vi "Main.vi"(4 "States":T1(ring), 5 "name":string="Name", 6 "error in":errorcluster, 8 "elemint in":variant, 9 "queue in":refnum<queue>) -> (0 "error out":errorcluster, 2 "element out":variant, 3 "queue out":refnum<queue>)   [LabVIEW 2010]
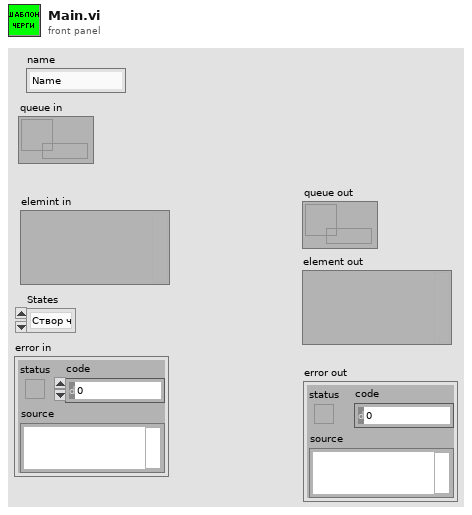
[diagram p1: front panel]
types:
  T1 = enum16{"Створ ч", "Зап на поч", "Зап на кін", "Зчит", "Очищ", "Видал"}
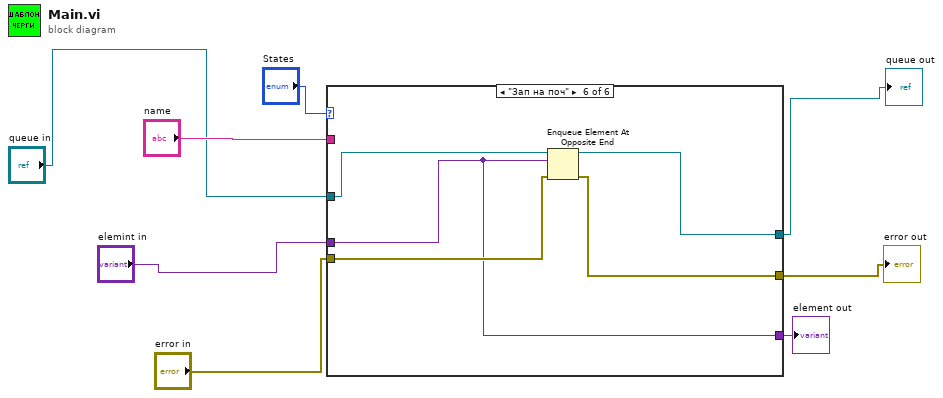
[diagram p0: block diagram]
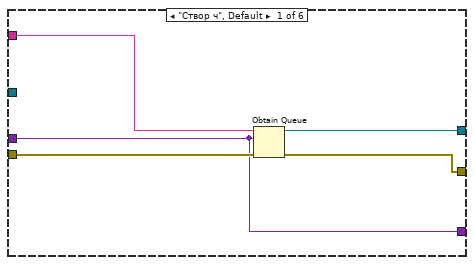
[diagram p2: hidden frame]
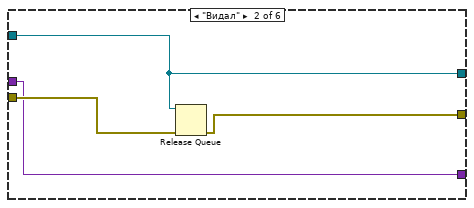
[diagram p3: hidden frame]
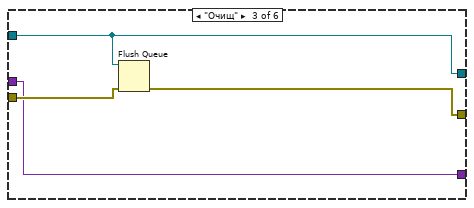
[diagram p4: hidden frame]
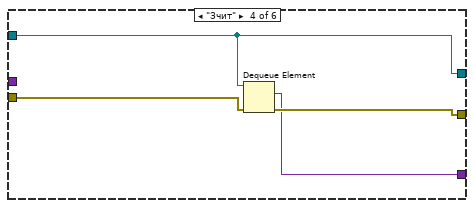
[diagram p5: hidden frame]
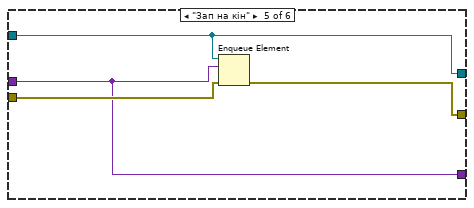
[diagram p6: hidden frame]
diagram:
  n1 = case shown="\"Зап на поч\"" "States" {
    tunnel: "name" -> [w13 _ _ _ _ _]
    tunnel: "elemint in" -> [w9 w14 w18 _ w26 w30]
    tunnel: [w12 w15 w19 w22 w27 w31] -> w3
    tunnel: [w11 w17 w21 w25 w29 w34] -> w6
    tunnel: "error in" -> [w10 w16 w20 w24 w28 w33]
    tunnel: "queue in" -> [_ w15 w19 w22 w27 w32]
    tunnel: [w9 w14 w18 w23 w26 w30] -> w1
    frame "Створ ч", Default {
      n2 = Obtain Queue(name (unnamed)=w13, element data type=w9, error in (no error)=w10) -> (queue out=w12:refnum<queue>, error out=w11:errorcluster)  [unwired: 2 in, 1 out]
    }
    frame "Видал" {
      n3 = Release Queue(queue=w15, error in (no error)=w16) -> (error out=w17:errorcluster)  [unwired: 1 in, 2 out]
    }
    frame "Очищ" {
      n4 = Flush Queue(queue=w19, error in (no error)=w20) -> (error out=w21:errorcluster)  [unwired: 2 out]
    }
    frame "Зчит" {
      n5 = Dequeue Element(queue=w22, error in (no error)=w24) -> (element=w23:variant, error out=w25:errorcluster)  [unwired: 1 in, 2 out]
    }
    frame "Зап на кін" {
      n6 = Enqueue Element(queue=w27, element=w26, error in (no error)=w28) -> (error out=w29:errorcluster)  [unwired: 1 in, 2 out]
    }
    frame "Зап на поч" {
      n7 = Enqueue Element At Opposite End(queue=w32, element=w30, error in (no error)=w33) -> (queue out=w31:refnum<queue>, error out=w34:errorcluster)  [unwired: 1 in, 1 out]
    }
  }
  "error out" <- w6
  "queue out" <- w3
  "element out" <- w1
